vi "Main.vi"() -> ()   [LabVIEW 2018]
panel:
  in  "Tab Control":enum32{"改变位图", "置反阈值", "颜色识别", "数字识别"}(tab)
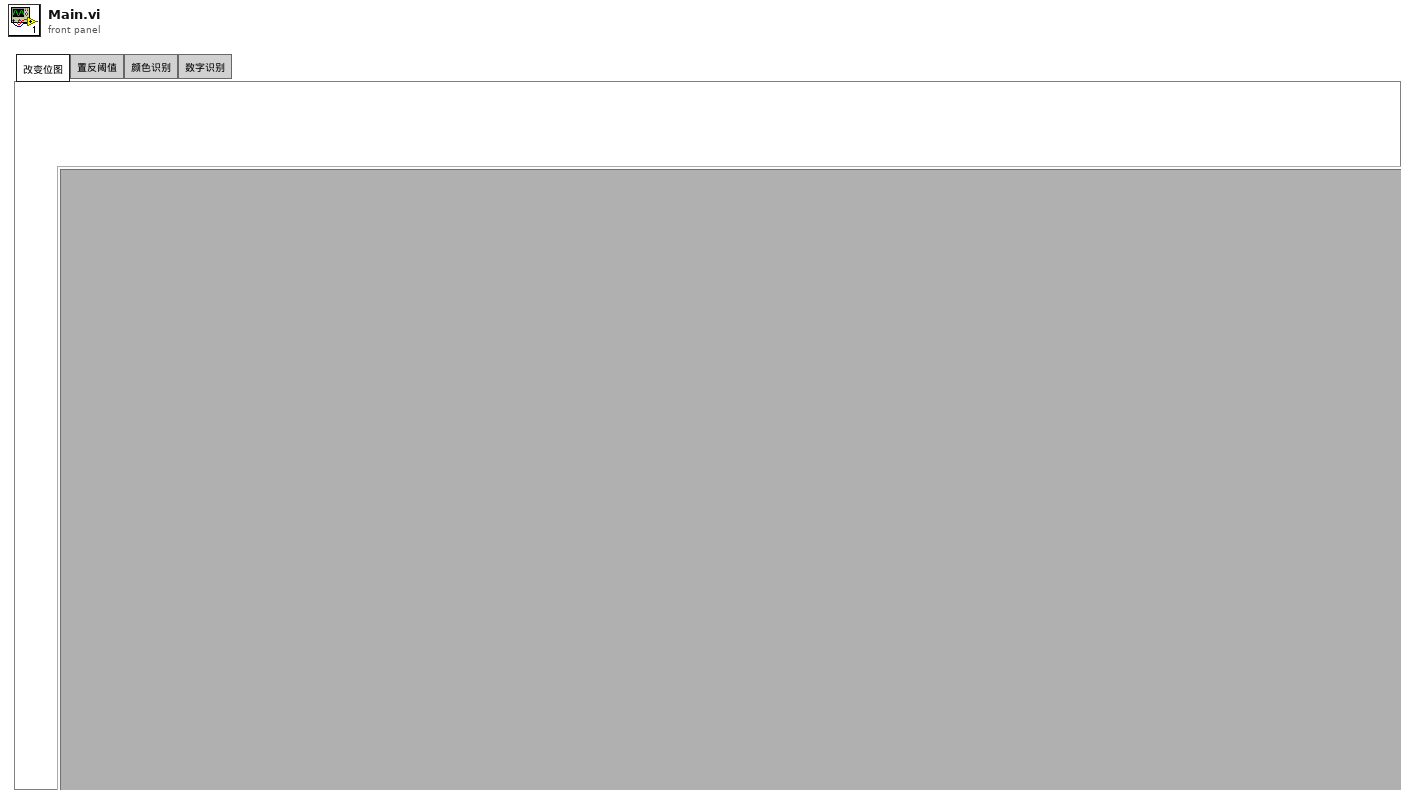
[diagram p1: front panel]
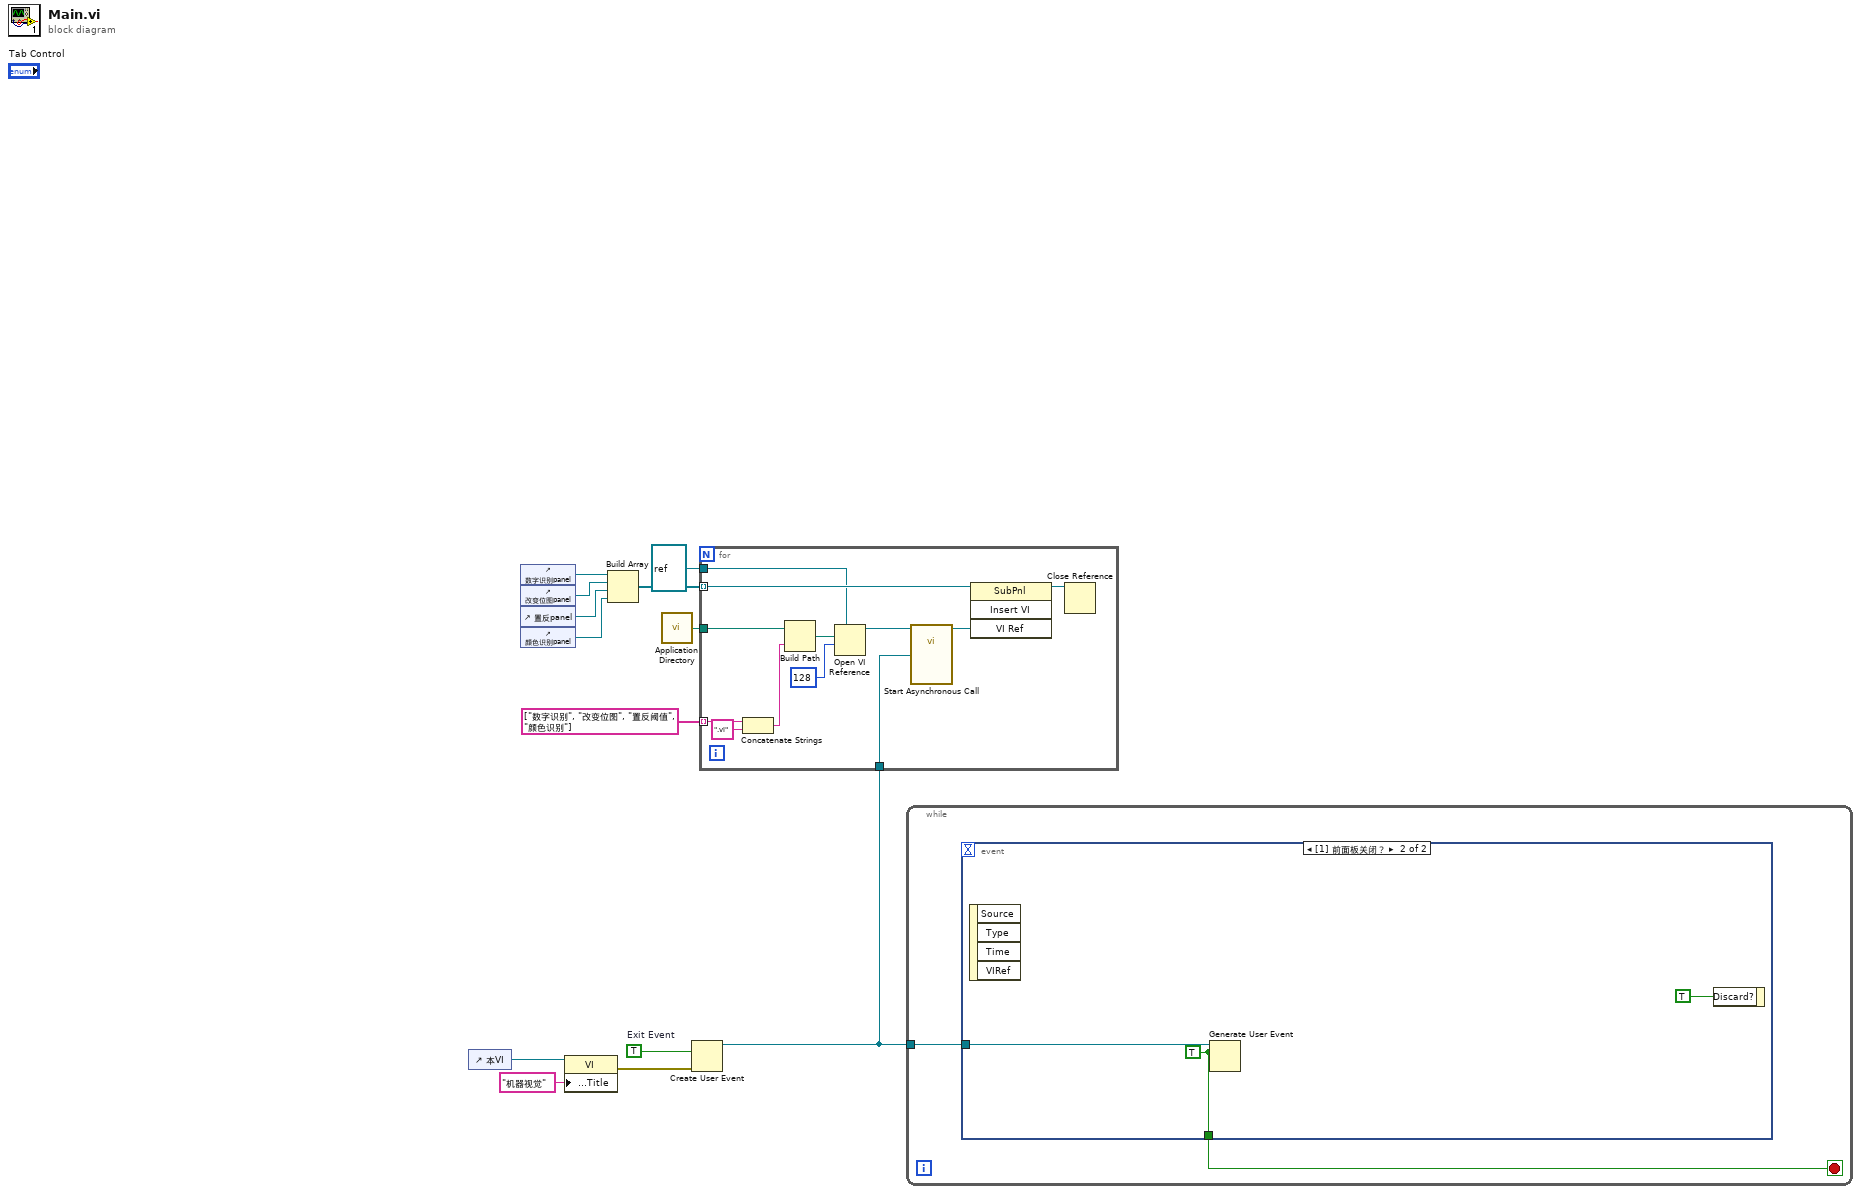
[diagram p0: block diagram]
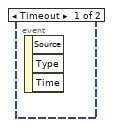
[diagram p2: hidden frame]
diagram:
  w13 = TRUE  # Exit Event
  n1 = control-ref of="本VI"() -> (w3:refnum<vi>)
  n2 = control-ref of="数字识别panel"() -> (w11:refnum<vi>)
  n3 = control-ref of="改变位图panel"() -> (w10:refnum<vi>)
  n4 = control-ref of="置反panel"() -> (w9:refnum<vi>)
  n5 = control-ref of="颜色识别panel"() -> (w8:refnum<vi>)
  n6 = property class="VI"(reference=w3, "Front Panel.Title"="机器视觉" ("VI名称")) -> (error out=w1:errorcluster)  [unwired: 1 in, 1 out]
  n7 = Build Array(w11, w10, w9, w8) -> (w7:refnum<vi>[])
  n8 = call <vilib>:"Application Directory.vi"() -> ("Application Directory"=w6:path)
  n9 = Create User Event(user event datatype=w13, error in=w1) -> (user event=w12:refnum<user-event>)  [unwired: 1 out]
  n10 = for {
    tunnel: w12 -> [w22]
    tunnel: w7 -> [w20] mode=indexing
    tunnel: w6 -> [w19]
    tunnel: string[] ["数字识别", "改变位图", "置反阈值", "颜色识别"] -> [w18] mode=indexing
    tunnel: refnum<vi> refnum ("type specifier VI Refnum (for type only)") -> [w14]
    n11 = Concatenate Strings(w18, ".vi" ("string")) -> (w16:string)
    n12 = Build Path(base path=w19, name or relative path=w16) -> (appended path=w15:path)
    n13 = Open VI Reference(type specifier VI Refnum (for type only)=w14, vi path=w15, options=128) -> (vi reference=w25:refnum<vi>)  [unwired: 3 in, 1 out]
    n14 = call-by-ref "Start Asynchronous Call"(reference=w25, "Exit Event"=w22) -> (reference out=w24:refnum<vi>)  [unwired: 3 in, 1 out]
    n15 = invoke class="SubPnl" method="Insert VI"(reference=w20, "VI Ref"=w24) -> (reference out=w23:refnum<vi>)  [unwired: 2 in, 3 out]
    n16 = Close Reference(reference=w23) -> ()  [unwired: 1 in, 1 out]
  }
  n17 = while {
    tunnel: w12 -> [w27]
    stop <- w26 stop-if-true
    n18 = event shown="[1] 前面板关闭？" {
      selector: _ -> [_ _]
      dyn-events: _ -> [_ _]
      timeout: _ -> [_ _]
      tunnel: w27 -> [_ w30]
      tunnel: [_ w29] -> w26
      event Timeout {
        n19 = event-data() -> ()  [unwired: 1 in, 3 out]
      }
      event Panel Close? {
        w29 = TRUE ("event data")
        n20 = event-data() -> ()  [unwired: 1 in, 4 out]
        n21 = Generate User Event(user event=w30, event data cluster=w29) -> ()  [unwired: 2 in, 2 out]
        n22 = event-data("Discard?"=TRUE) -> ()  [unwired: 1 in, 1 out]
      }
    }
  }
